vi "Server Handle Configure Write Message.vi"(7 "port":u16, 8 "error in":errorcluster, 9 "data string":string, 10 "connection info in":T1, 11 "state in":T3) -> (0 "error out":errorcluster, 3 "state out":T3)   [LabVIEW 2010, in "NI_CCC.lvlib"]
uses:
  NI_CCC.lvlib
  Server State.ctl
  <vilib>/NI/STM/TCP/TCP Connection Info.ctl
  <vilib>/NI/STM/SubVIs/MetaDataElement.ctl
  <vilib>/NI/STM/NI STM.lvlib
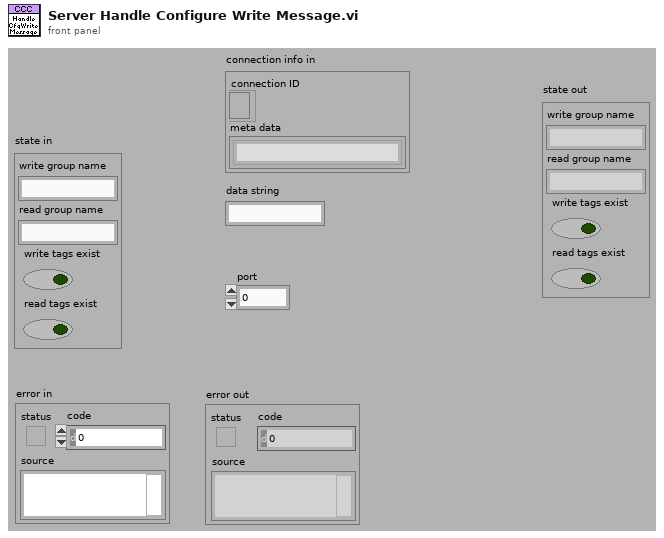
[diagram p1: front panel]
types:
  T1 = typedef "NI STM.lvlib/TCP Connection Info.ctl" = cluster{"connection ID":refnum<k5>, "meta data":T2[]}
  T2 = typedef "NI STM.lvlib/MetaDataElement.ctl" = string
  T3 = typedef "NI_CCC.lvlib/Server State.ctl" = cluster{"write group name":string, "read group name":string, "write tags exist":bool, "read tags exist":bool}
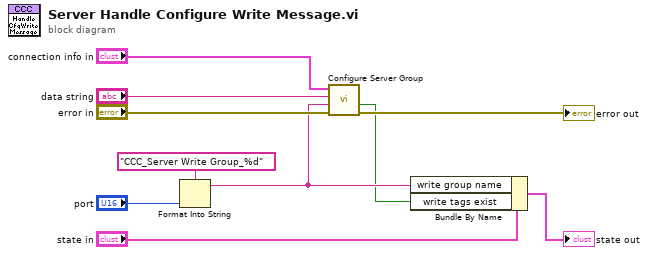
[diagram p0: block diagram]
diagram:
  n1 = Format Into String(format string="CCC_Server Write Group_%d", "port") -> (resulting string=w3:string)  [unwired: 2 in, 1 out]
  n2 = call "Configure Server Group.vi"("error in"="error in", "group name"=w3, "data string"="data string", "connection info in"="connection info in") -> ("error out"=→"error out":errorcluster, "tags exist?"=w1:bool)  [unwired: 6 in]
  n3 = Bundle By Name(cluster="state in", "write group name"=w3, "write tags exist"=w1) -> (→"state out":T3)
